vi "UsrProfiles-Window-About.vi"   [LabVIEW 2013]
doc: "Use this template to create a dialog box with event handling."
uses:
  <vilib>/Utility/miscctls.llb/LVPointTypeDef.ctl
  Global Variables/General Globals.vi
panel:
  # "Use this window to create your own software setup profiles to avoid interfering with other people's setup and prevent others changing your personal settings.\n\nYou can create any number of profiles under your own user account. \n\nRight-click on the profiles list to view profile management options."
types:
  T1 = typedef "LVPointTypeDef.ctl" = cluster{"Horizontal":i16, "Vertical":i16}
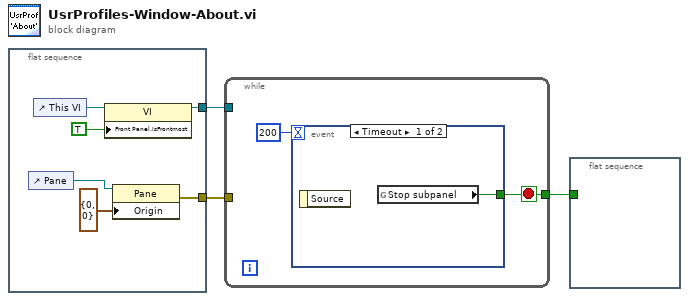
[diagram p0: block diagram]
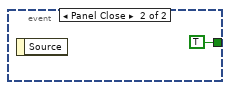
[diagram p2: hidden frame]
diagram:
  n1 = flat-sequence {
    tunnel: [w7] -> w3
    tunnel: [w5] -> w2
    frame #0 {
      n2 = control-ref of="Pane"() -> (w4:refnum<vi>)
      n3 = control-ref of="This VI"() -> (w8:refnum<vi>)
      n4 = property on="Property Node" class="VI"(reference=w8, "Front Panel.IsFrontmost"=TRUE ("Front Panel Window:Is Frontmost")) -> (reference out=w7:refnum<vi>)  [unwired: 1 in, 1 out]
      n5 = property class="Pane"(reference=w4, "Origin"=T1 {"Horizontal"=0, "Vertical"=0}) -> (error out=w5:errorcluster)  [unwired: 1 in, 1 out]
    }
  }
  n6 = while {
    tunnel: w2 -> [_]
    tunnel: w3 -> [_]
    tunnel: [w10] -> w1
    stop <- w10 stop-if-true
    n7 = event shown="[0] Timeout" {
      selector: _ -> [_ _]
      dyn-events: _ -> [_ _]
      timeout: 200 -> [_ _]
      tunnel: [w12 TRUE ("Stop?")] -> w10
      event Timeout {
        n8 = event-data() -> ()  [unwired: 1 in, 1 out]
        n9 = global read "General Globals.vi" "Stop subpanel"() -> (w12:bool)
      }
      event Panel Close {
        n10 = event-data() -> ()  [unwired: 1 in, 1 out]
      }
    }
  }
  n11 = flat-sequence {
    tunnel: w1 -> [_]
    frame #0 {
    }
  }
